vi "measurement_configurator.vi"() -> ()   [LabVIEW 2015]
doc: "Copyright (c) 2018 Frans Korhonen, Institute for Atmospheric and Earth System Research / Physics, Faculty of Science, University of Helsinki, Finland\n\nThis file is part of MeasGUI.\n\nThis Source Code Form is subject to the terms of the Mozilla Public\nLicense, v. 2.0. If a copy of the MPL was not distributed with this\n file, You can obtain one at http://mozilla.org/MPL/2.0/."
panel:
  in  "file cluster":T1={"open program folder"=FALSE, "Load"=FALSE, "Save"=FALSE, "Saved Configuration"="default", "output filename"="measurement.bat", "output"=FALSE}
  out "program path":path
  out "saved controls":string[](array[string])=["measurement channels", "measurement comments", "measurement parameters", "measurement settings", "measurement logging", "connection settings", "X channel", "Y channels", "Log x", "Log y", "save measurement", "measurement start commands", "measurement end commands"]
  in  "Tab Control":T2(tab)=enum."flowmeters"
  in  "serial device update rate":dbl=1.0
  in  "Serial devices":T3(array[cluster])
  in  "scaled output":T4(array[cluster])
  in  "scaled input":T5(array[cluster])
  in  "Electometer scaling":T6(array[cluster])
  in  "Concentration counters":T7(array[cluster])
  in  "TSI flowmeters":T8(array[cluster])
  in  "PID controllers":T9(array[cluster])
  in  "loggers":T10(array[cluster])
  in  "postconfiguration":string="#postconfiguration"
  in  "preconfiguration":string="create pipeserver pipe\nsetup pipe \"\\\\.\\pipe\\channel_system\"\nlink pipe control\n\nread control hardware.ini"
  out "configuration":string
  # "factor=current[A]/input"
  # "Will also create:\n\"channel_name\"_flow\n\"channel_name\"_t\n\"channel_name\"_p\n\nchannels for different measured parameters"
  # "Time specifiers in filenames \n%Y=year\n%m=Month as number\n%d = Day of the month\n%H =Hour in 24h format\n%M =Minute\n%S = seconds\n%z = Timezone offset"
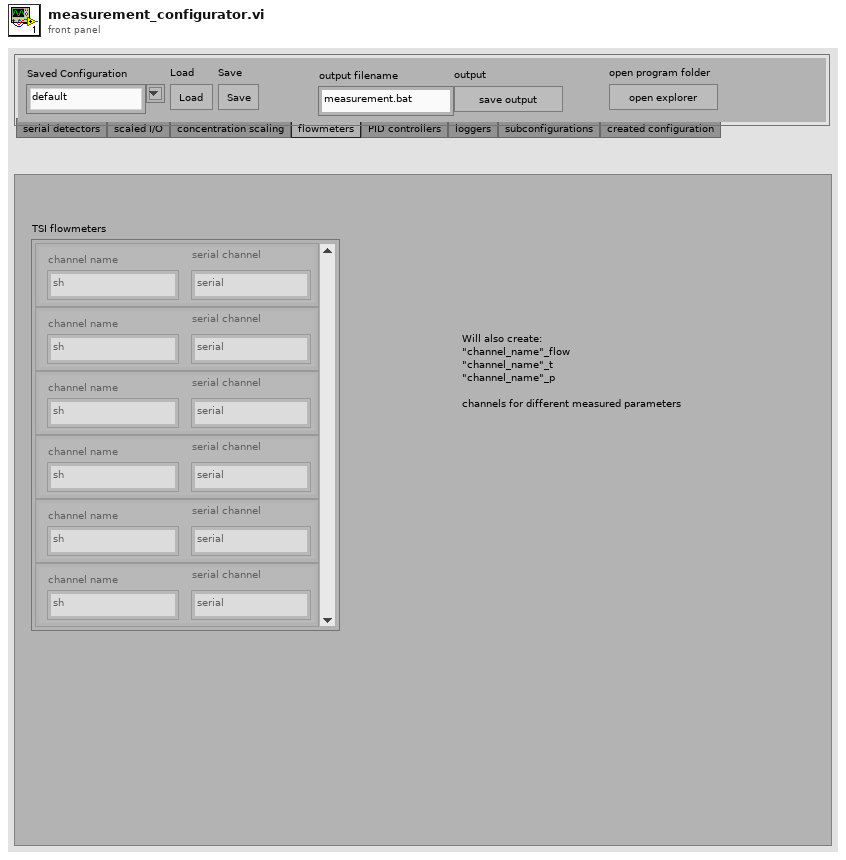
[diagram p1: front panel]
types:
  T1 = cluster{"open program folder":bool, "Load":bool, "Save":bool, "Saved Configuration":string, "output filename":string, "output":bool}
  T2 = enum32{"serial detectors", "scaled I/O", "concentration scaling", "flowmeters", "PID controllers", "loggers", "subconfigurations", "created configuration"}
  T3 = cluster{"channel name":string, "serial channel":string, "device":enum16{"Airmodus CPC", "TSI CPC", "TSI Electrometer", "Keithley EM", "TSI water CPC", "TSI CPC 3010"}}[]
  T4 = cluster{"channel name":string, "in 1":dbl, "output channel":string, "out 1":dbl, "in 2":dbl, "out 2":dbl}[]
  T5 = cluster{"channel name":string, "in 1":dbl, "input channel":string, "out 1":dbl, "in 2":dbl, "out 2":dbl}[]
  T6 = cluster{"channel name":string, "sample flow":dbl, "input channel":string, "factor":dbl, "input offset":dbl}[]
  T7 = cluster{"channel name":string, "sample flow":dbl, "counter input channel":string}[]
  T8 = cluster{"channel name":string, "serial channel":string}[]
  T9 = cluster{"channel name":string, "P":dbl, "input channel":string, "I":dbl, "in min":dbl, "in max":dbl, "out max":dbl, "out min":dbl, "initial sepoint":dbl, "D":dbl, "controlled channel":string}[]
  T10 = cluster{"channel name":string, "filename":string, "name change interval [s]":u32, "channels to log":string[], "delimiter char":string, "trigger char":string, "input channel\nor log interval [s]":string}[]
  T11 = enum16{"open", "replace", "create", "open or create", "replace or create", "replace or create with confirmation"}
  T12 = enum16{"Airmodus CPC", "TSI CPC", "TSI Electrometer", "Keithley EM", "TSI water CPC", "TSI CPC 3010"}
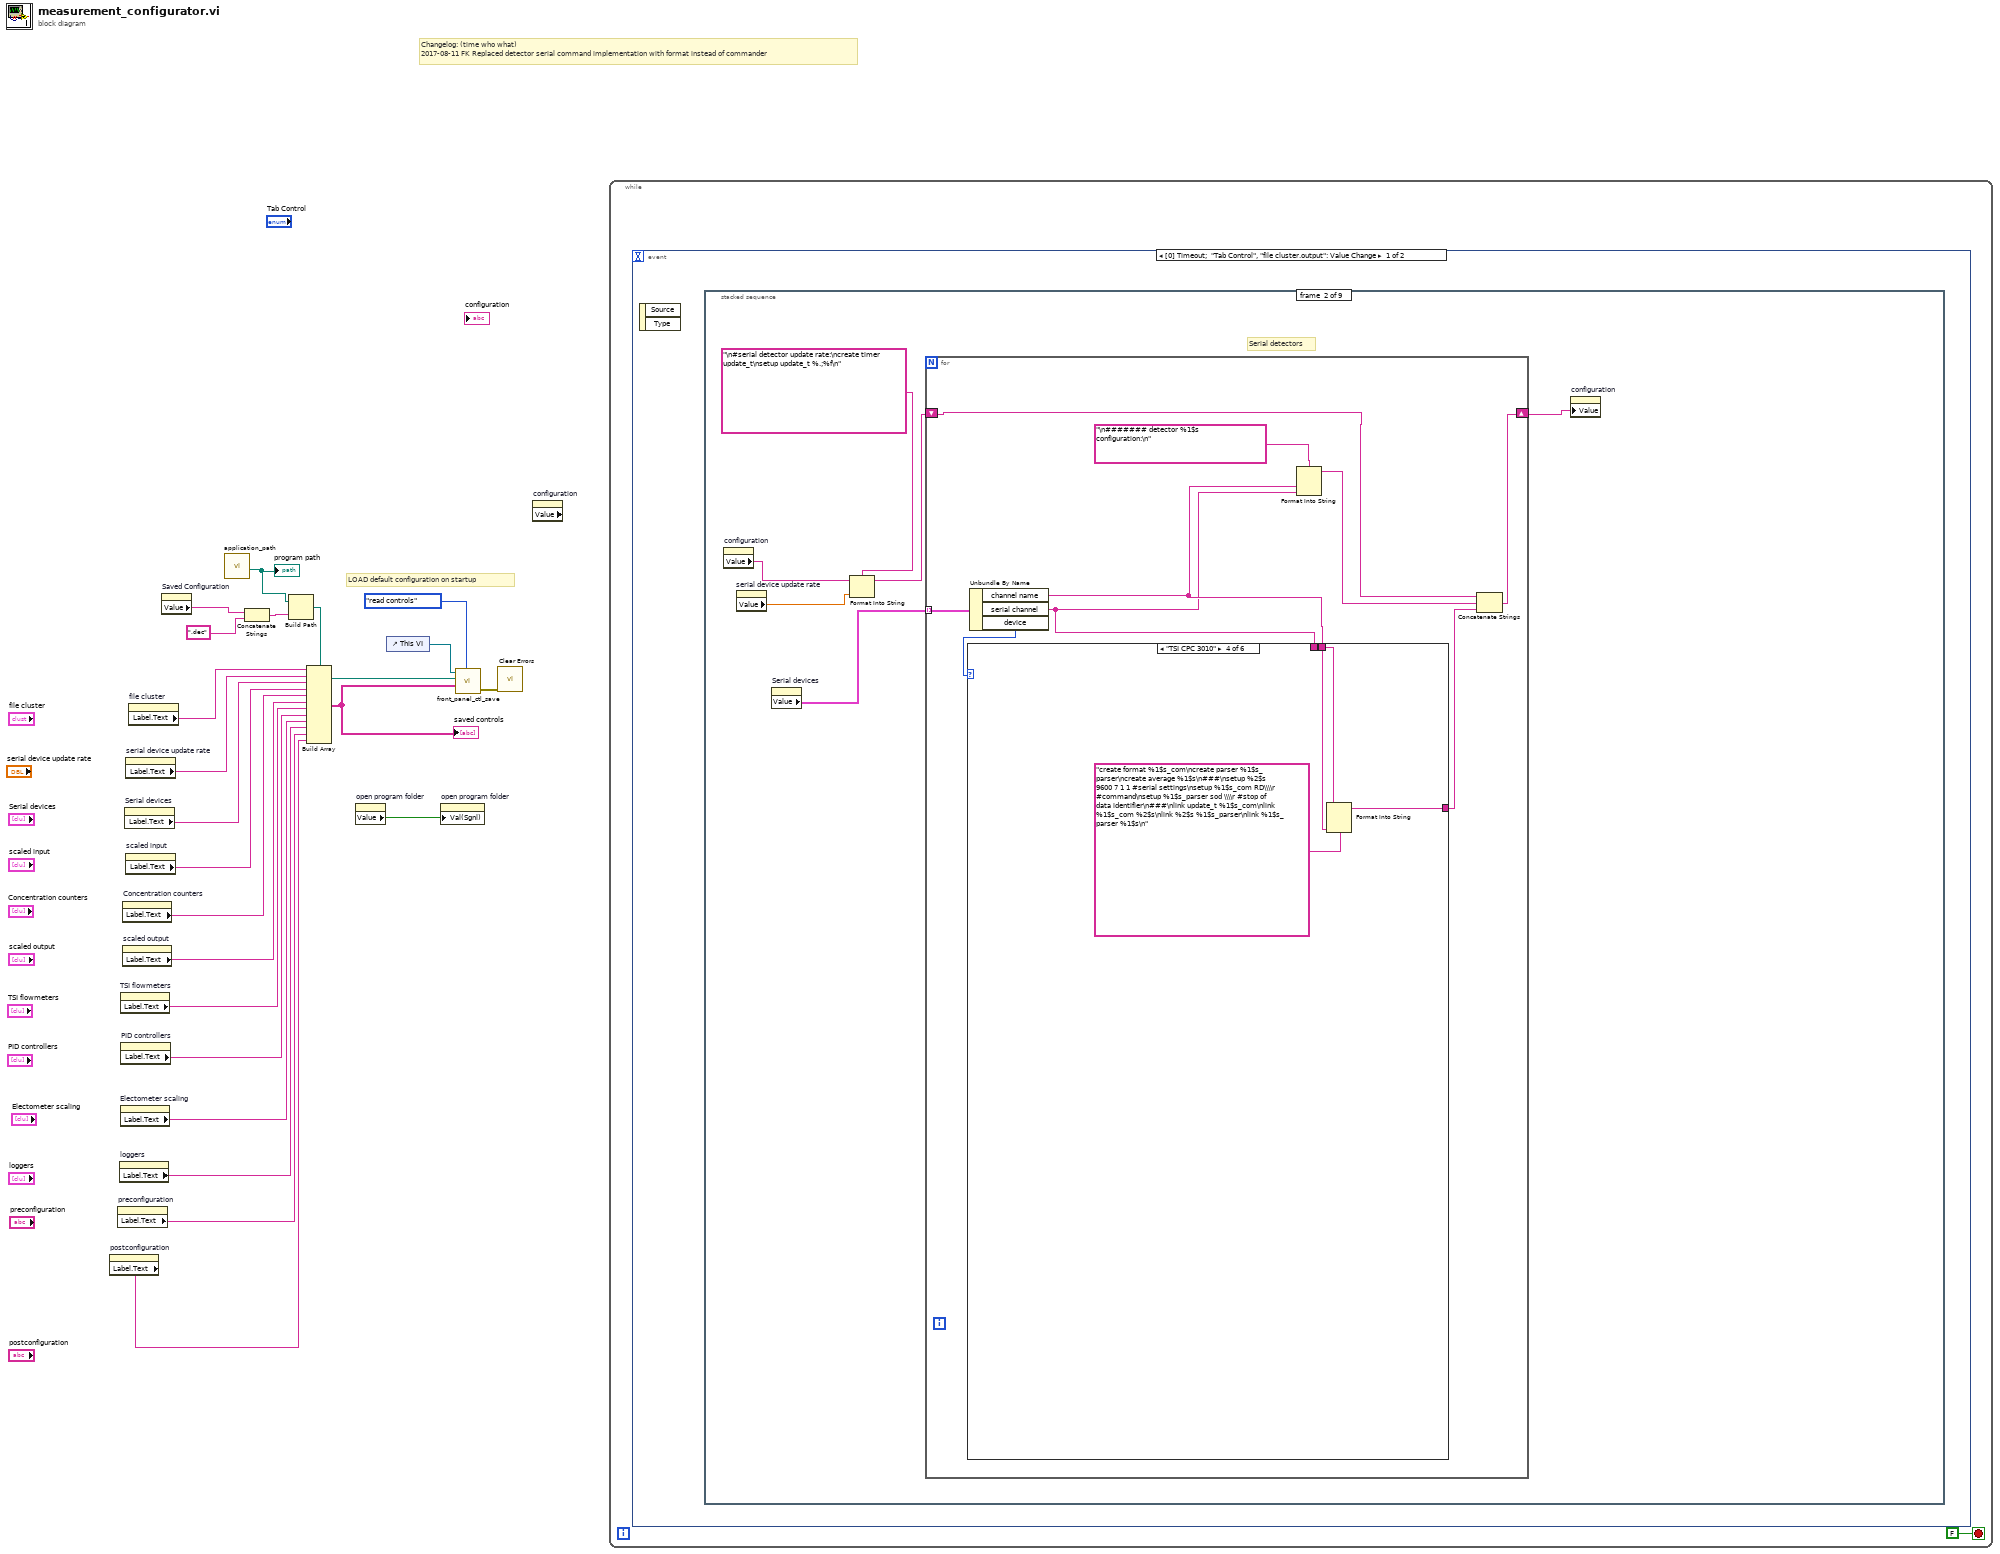
[diagram p0: block diagram]
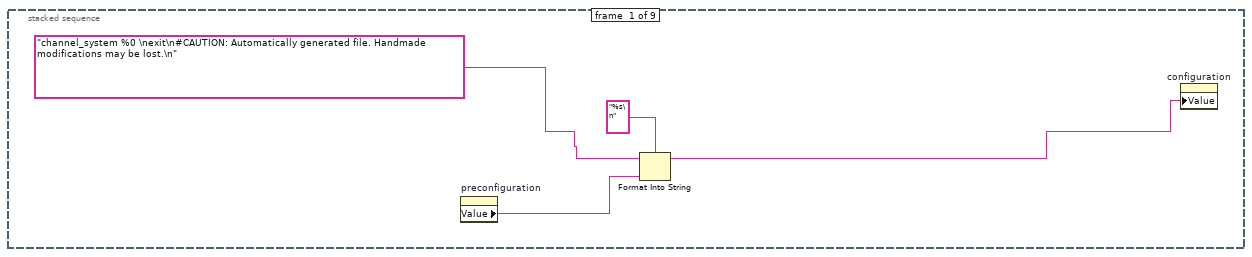
[diagram p2: hidden frame]
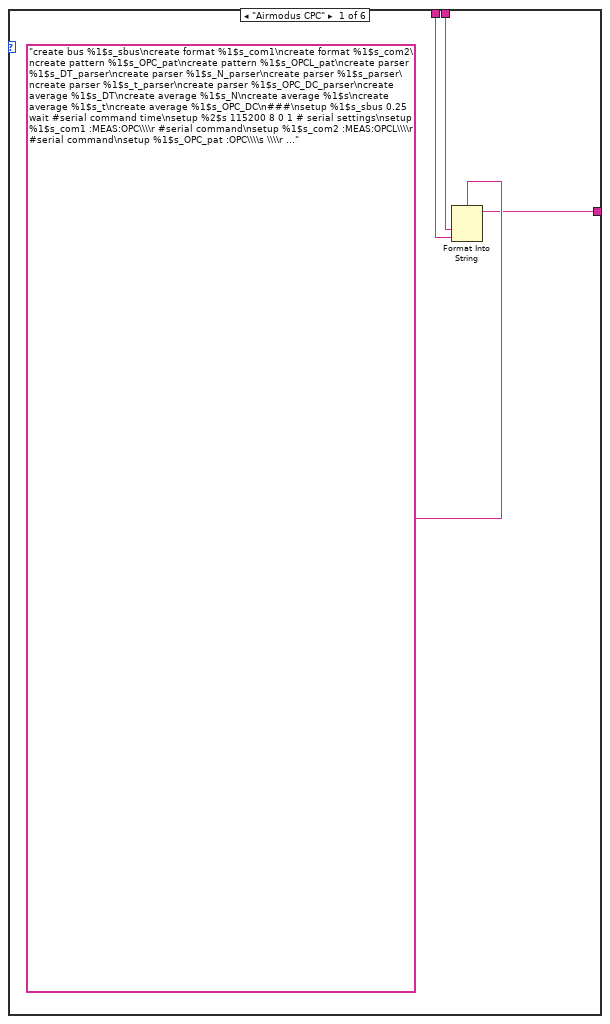
[diagram p3: hidden frame]
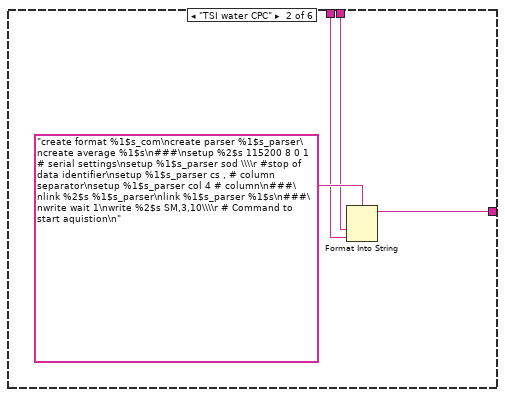
[diagram p4: hidden frame]
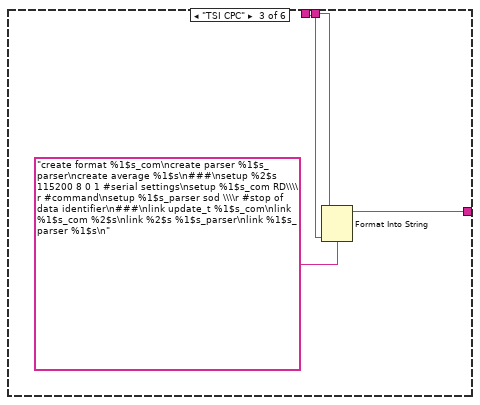
[diagram p5: hidden frame]
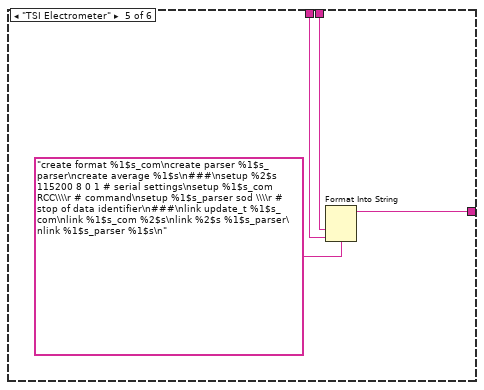
[diagram p6: hidden frame]
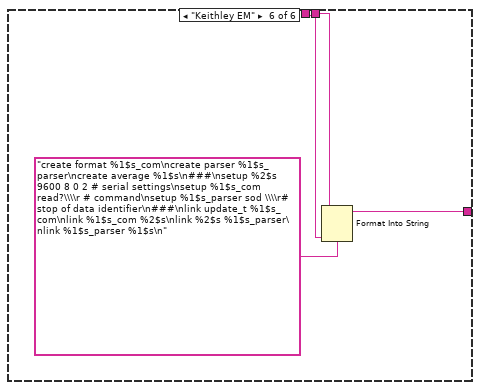
[diagram p7: hidden frame]
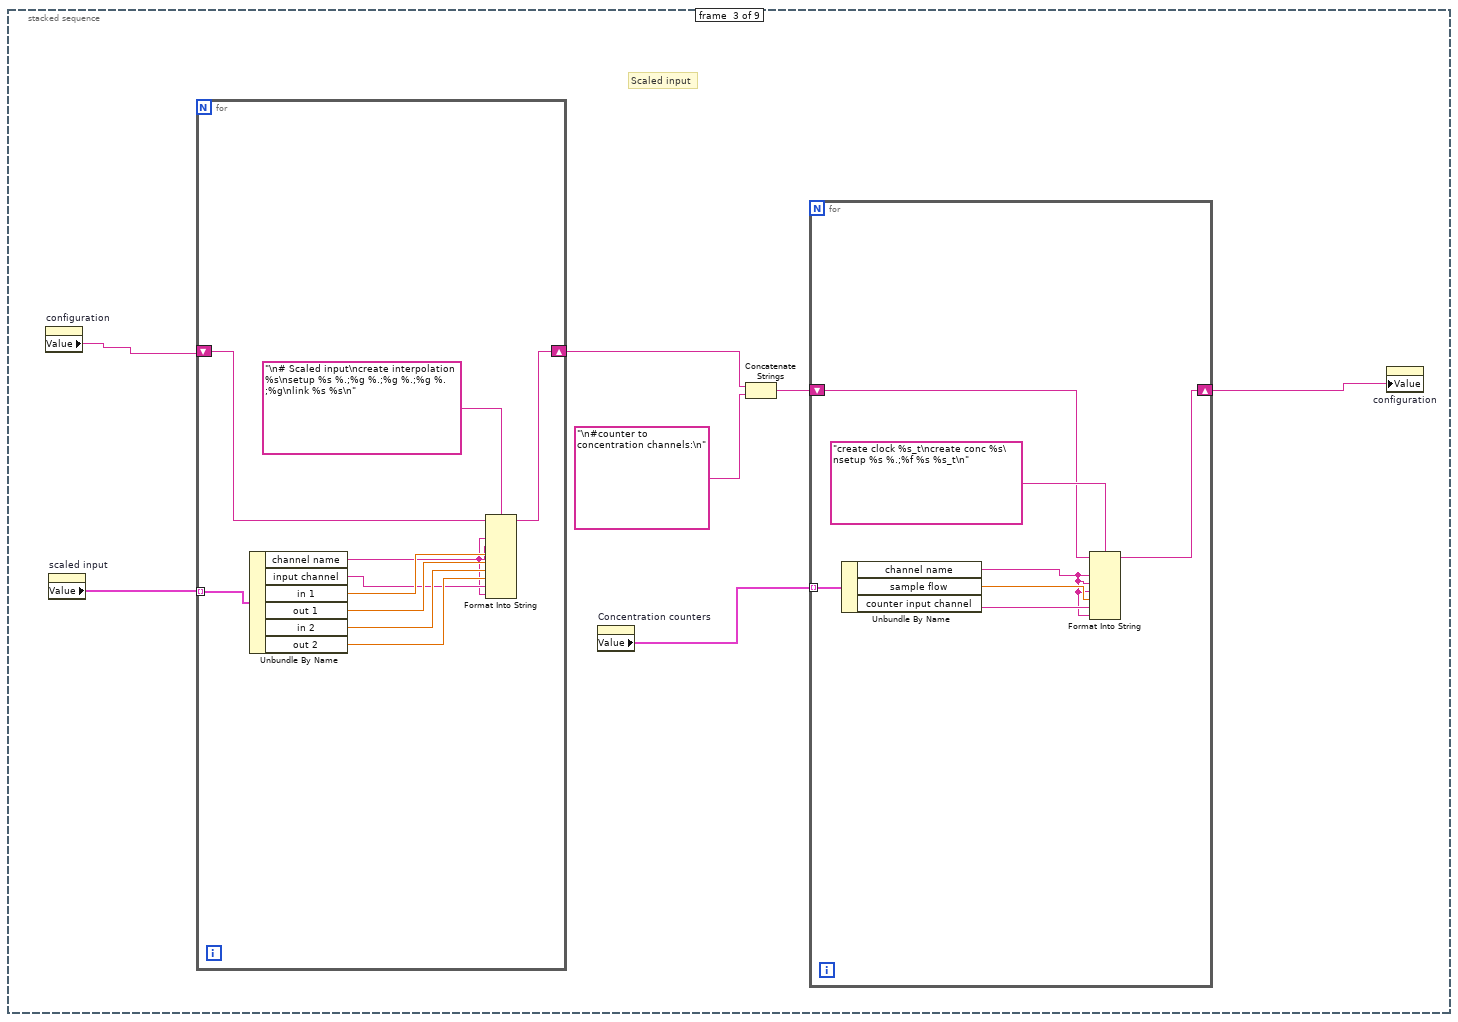
[diagram p8: hidden frame]
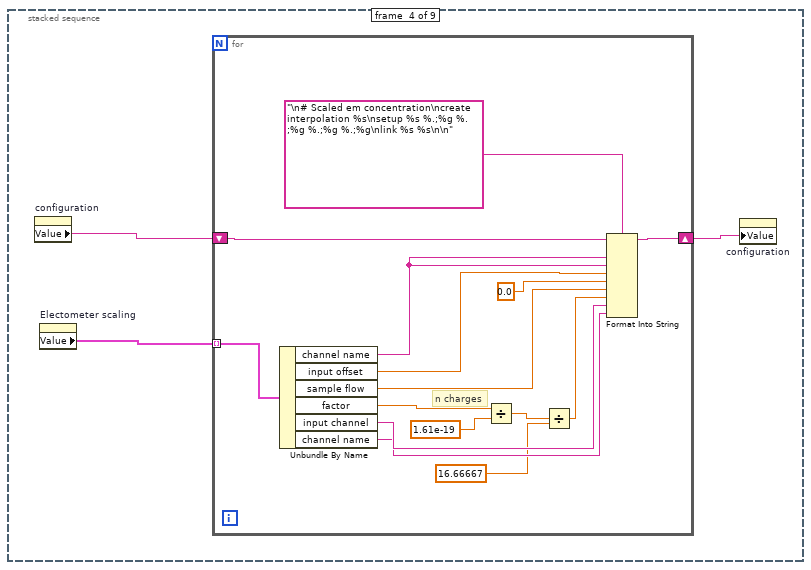
[diagram p9: hidden frame]
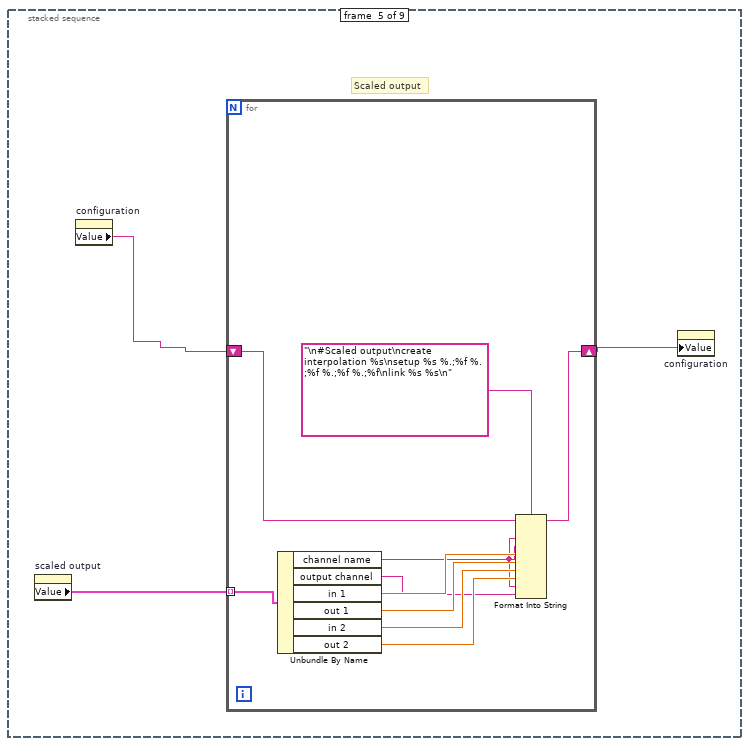
[diagram p10: hidden frame]
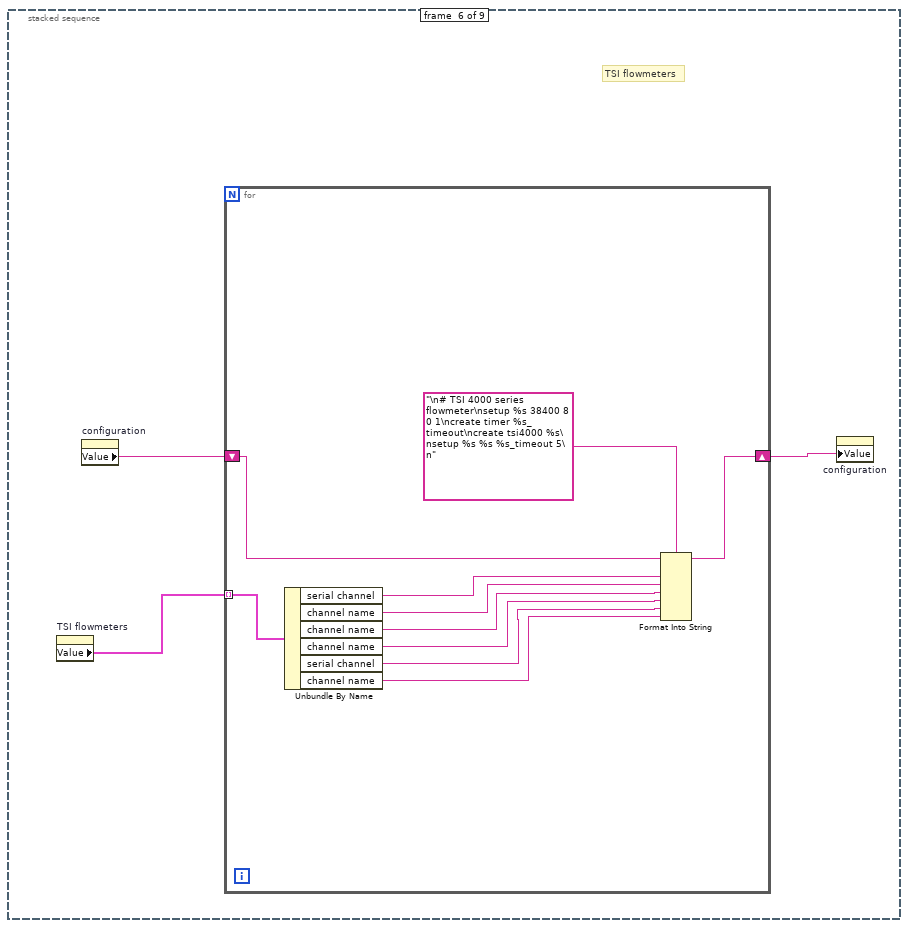
[diagram p11: hidden frame]
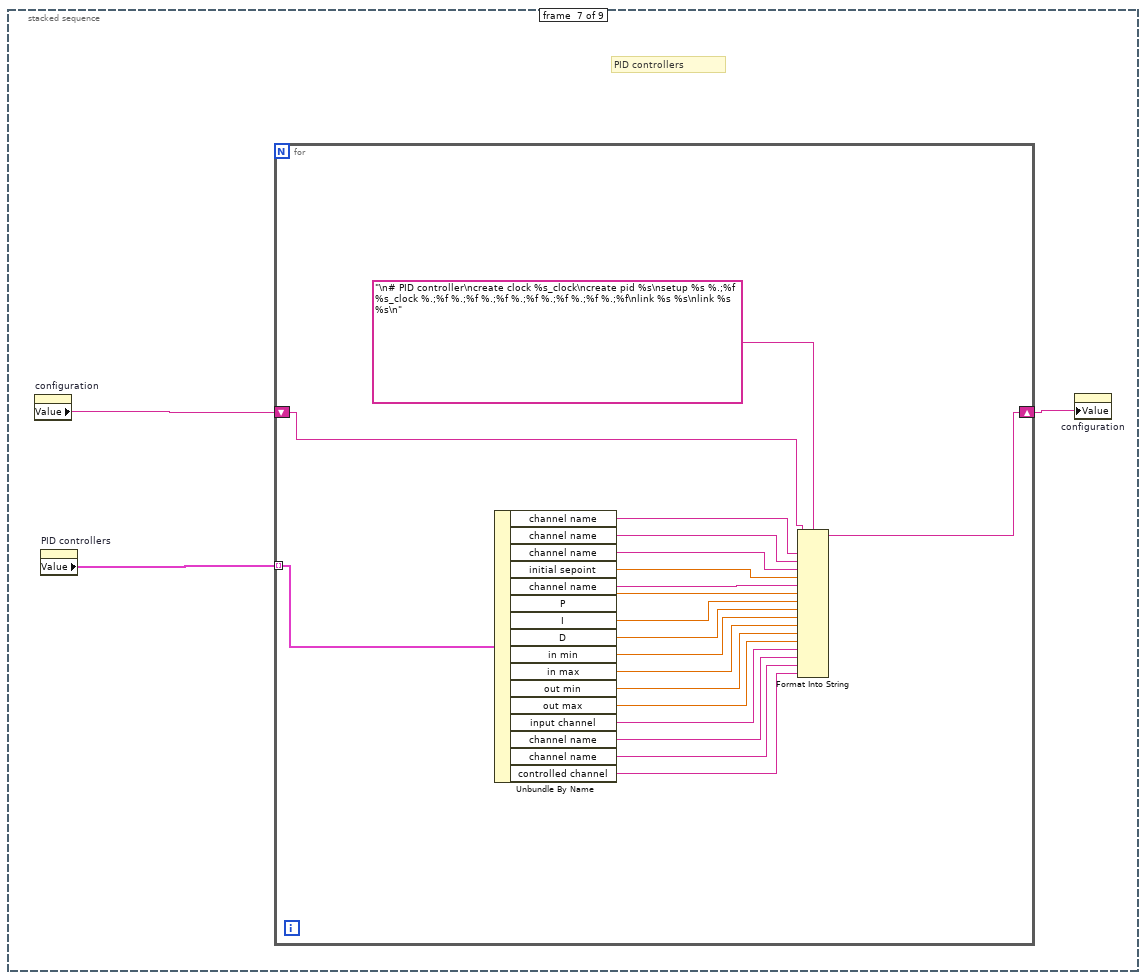
[diagram p12: hidden frame]
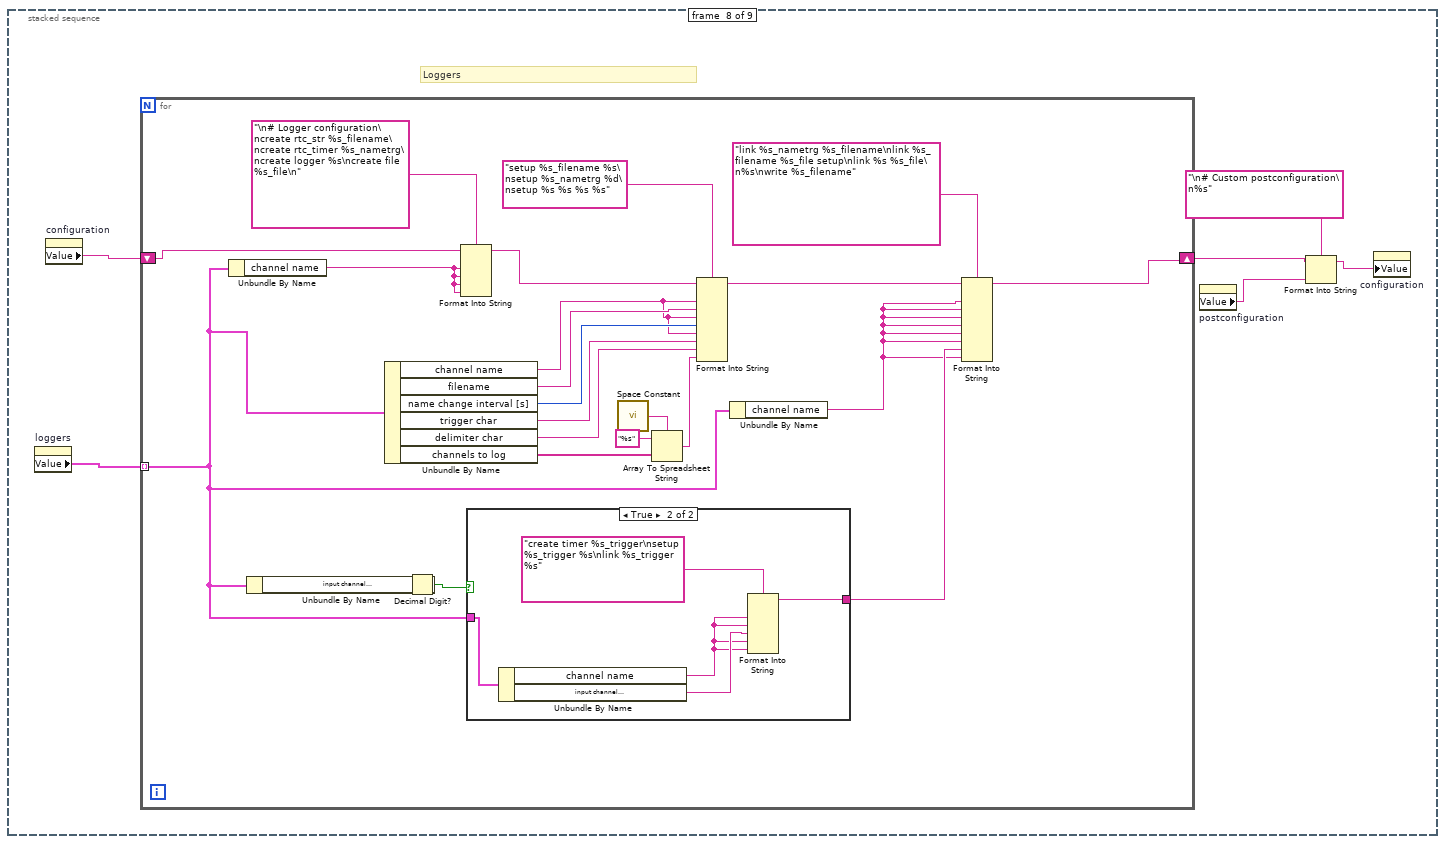
[diagram p13: hidden frame]
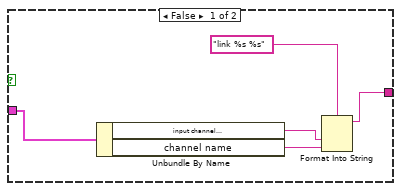
[diagram p14: hidden frame]
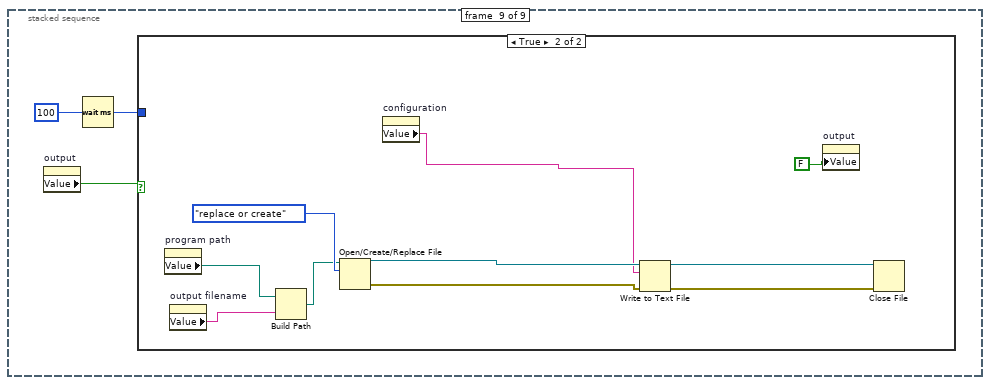
[diagram p15: hidden frame]
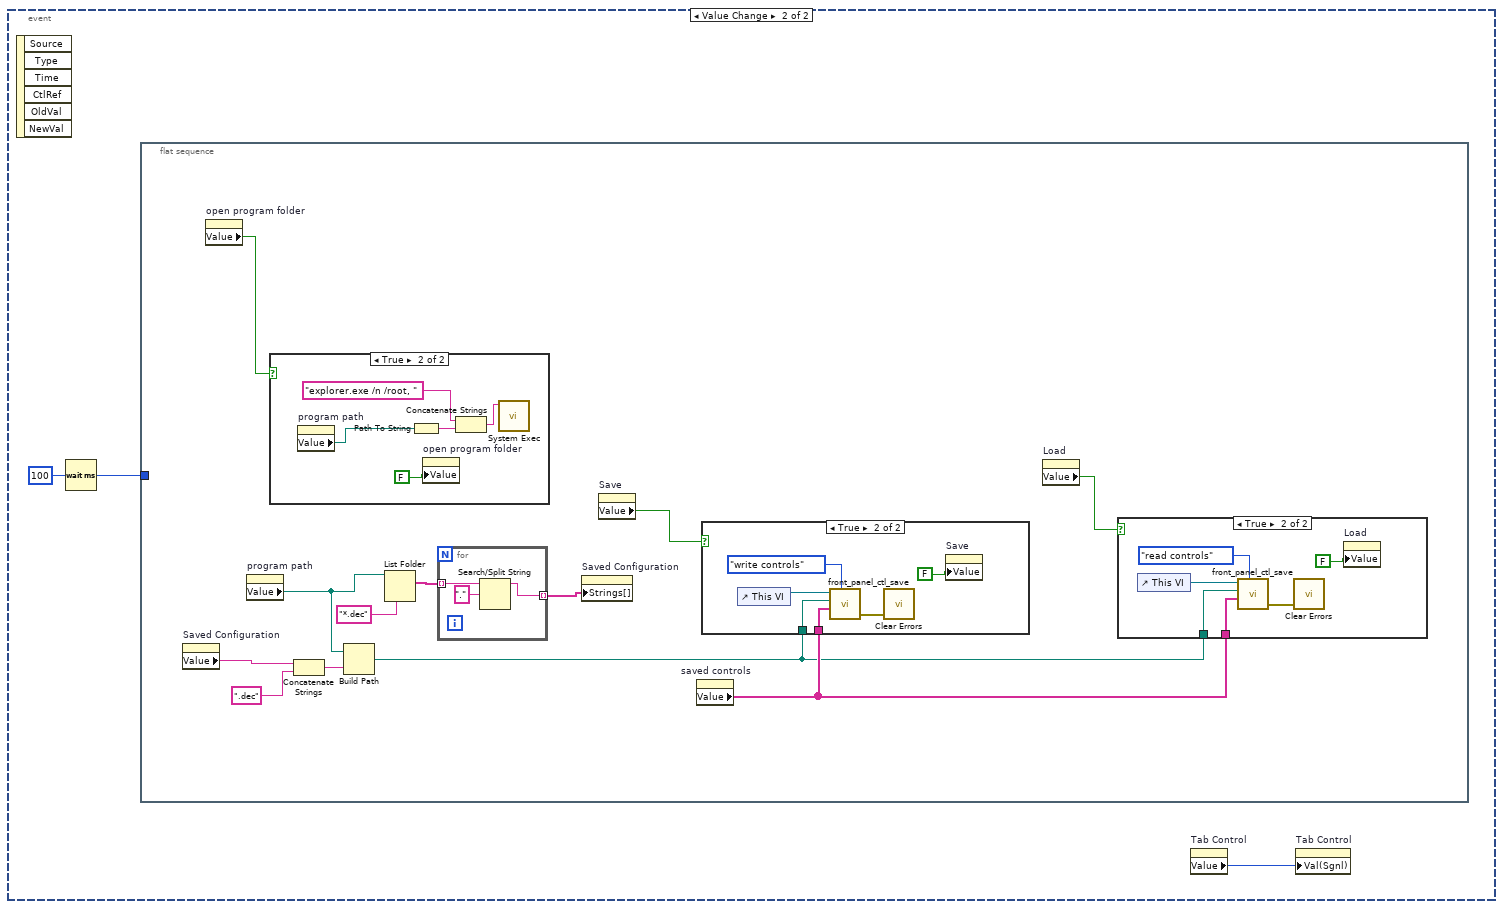
[diagram p17: hidden frame]
diagram:
  # "Changelog: (time who what)\n2017-08-11 FK Replaced detector serial command implementation with format instead of commander"
  # "LOAD default configuration on startup"
  n1 = property on="postconfiguration" class="Str"() -> ("Label.Text"=w1:string)  [unwired: 2 in, 2 out]
  n2 = property on="preconfiguration" class="Str"() -> ("Label.Text"=w2:string)  [unwired: 2 in, 2 out]
  n3 = property on="loggers" class="Arr (strict)"() -> ("Label.Text"=w4:string)  [unwired: 2 in, 2 out]
  n4 = property on="TSI flowmeters" class="Arr (strict)"() -> ("Label.Text"=w7:string)  [unwired: 2 in, 2 out]
  n5 = property on="Electometer scaling" class="Arr (strict)"() -> ("Label.Text"=w5:string)  [unwired: 2 in, 2 out]
  n6 = property on="PID controllers" class="Arr (strict)"() -> ("Label.Text"=w6:string)  [unwired: 2 in, 2 out]
  n7 = property on="Concentration counters" class="Arr (strict)"() -> ("Label.Text"=w12:string)  [unwired: 2 in, 2 out]
  n8 = property on="scaled output" class="Arr (strict)"() -> ("Label.Text"=w8:string)  [unwired: 2 in, 2 out]
  n9 = property on="Serial devices" class="Arr (strict)"() -> ("Label.Text"=w14:string)  [unwired: 2 in, 2 out]
  n10 = property on="serial device update rate" class="DigNum (strict)"() -> ("Label.Text"=w15:string)  [unwired: 2 in, 2 out]
  n11 = property on="scaled input" class="Arr (strict)"() -> ("Label.Text"=w13:string)  [unwired: 2 in, 2 out]
  n12 = property on="file cluster" class="Clust (strict)"() -> ("Label.Text"=w11:string)  [unwired: 2 in, 2 out]
  n13 = property on="Saved Configuration" class="CmbBox"() -> ("Value"=w17:string)  [unwired: 2 in, 2 out]
  n14 = call "application_path.vi"() -> ("path"=w10:path)  [unwired: 11 in]
  "program path" <- w10
  n15 = Concatenate Strings(w17, ".dec" ("string")) -> (w21:string)
  n16 = Build Path(base path=w10, name or relative path=w21) -> (appended path=w19:path)
  n17 = Build Array(w11, w15, w14, w13, w12, w8, w7, w6, w5, w4, w2, w1) -> (w16:string[])
  "saved controls" <- w16
  n18 = property on="open program folder" class="Bool (strict)"() -> ("Value"=w9:bool)  [unwired: 2 in, 2 out]
  n19 = control-ref of="This VI"() -> (w18:refnum<vi>)
  n20 = property on="open program folder" class="Bool (strict)"("Val(Sgnl)"=w9) -> ()  [unwired: 2 in, 2 out]
  n21 = call "front_panel_ctl_save.vi"("VI in"=w18, "method"=enum16{"read controls", "write controls"}."read controls", "filename"=w19, "controls"=w16) -> ("error out"=w3:errorcluster)  [unwired: 4 in]
  n22 = call <vilib>:"Clear Errors.vi"("error in (no error)"=w3) -> ()  [unwired: 5 in, 2 out]
  n23 = property on="configuration" class="Str" props=["Value"]() -> ()  [unwired: 2 in, 3 out]
  n24 = while {
    stop <- FALSE stop-if-true
    n25 = event shown="[0] Timeout;  \"Tab Control\", \"file cluster.output\": Value Change" {
      selector: _ -> [_ _]
      dyn-events: _ -> [_ _]
      timeout: _ -> [_ _]
      event Timeout; "Tab Control", "file cluster.output": Value Change {
        n26 = event-data() -> ()  [unwired: 1 in, 2 out]
        n27 = stacked-sequence {
          frame #0 {
            n28 = property on="preconfiguration" class="Str"() -> ("Value"=w27:string)  [unwired: 2 in, 2 out]
            n29 = Format Into String(format string="%s\n", initial string="channel_system %0 \nexit\n#CAUTION: Automatically generated file. Handmade modifications may be lost.\n", w27) -> (resulting string=w26:string)  [unwired: 1 in, 1 out]
            n30 = property on="configuration" class="Str"("Value"=w26) -> ()  [unwired: 2 in, 2 out]
          }
          frame #1 {
            # "Serial detectors"
            n31 = property on="configuration" class="Str"() -> ("Value"=w28:string)  [unwired: 2 in, 2 out]
            n32 = property on="serial device update rate" class="DigNum (strict)"() -> ("Value"=w29:dbl)  [unwired: 2 in, 2 out]
            n33 = property on="Serial devices" class="Arr (strict)"() -> ("Value"=w32:T3)  [unwired: 2 in, 2 out]
            n34 = Format Into String(format string="\n#serial detector update rate:\ncreate timer update_t\nsetup update_t %.;%f\n", initial string=w28, w29) -> (resulting string=w30:string)  [unwired: 1 in, 1 out]
            n35 = for {
              tunnel: w32 -> [w42] mode=indexing
              shift-right: [w38] -> w33
              shift-left: w30 -> [w37]
              n36 = Unbundle By Name(w42) -> ("channel name"=w35:string, "serial channel"=w34:string, "device"=w36:T12)
              n37 = case shown="\"TSI CPC 3010\"" w36 {
                tunnel: w34 -> [w43 w47 w51 w55 w59 w63]
                tunnel: [w45 w50 w53 w57 w61 w65] -> w39
                tunnel: w35 -> [w44 w48 w52 w56 w60 w64]
                frame "Airmodus CPC" {
                  n38 = Format Into String(format string="create bus %1$s_sbus\ncreate format %1$s_com1\ncreate format %1$s_com2\ncreate pattern %1$s_OPC_pat\ncreate pattern %1$s_OPCL_pat\ncreate parser %1$s_DT_parser\ncreate parser %1$s_N_parser\ncreate parser %1$s_parser\ncreate parser %1$s_t_parser\ncreate parser %1$s_OPC_DC_parser\ncreate average %1$s_DT\ncreate average %1$s_N\ncreate average %1$s\ncreate average %1$s_t\ncreate average %1$s_OPC_DC\n###\nsetup %1$s_sbus 0.25 wait #serial command time\nsetup %2$s 115200 8 0 1 # serial settings\nsetup %1$s_com1 :MEAS:OPC\\\\r #serial command\nsetup %1$s_com2 :MEAS:OPCL\\\\r  #serial command\nsetup %1$s_OPC_pat :OPC\\\\s \\\\r 256\nsetup %1$s_OPCL_pat :OPCL\\\\s \\\\r 256\n###\nsetup %1$s_DT_parser sod \\\\r #stop of data identifier\nsetup %1$s_DT_parser cs , # column separator\nsetup %1$s_DT_parser col 0 # column\n###\nsetup %1$s_N_parser sod \\\\r #stop of data identifier\nsetup %1$s_N_parser cs , # column separator\nsetup %1$s_N_parser col 1 # column\n###\nsetup %1$s_parser sod \\\\r #stop of data identifier\nsetup %1$s_parser cs , # column separator\nsetup %1$s_parser col 2 # column\n###\nsetup %1$s_t_parser sod \\\\r #stop of data identifier\nsetup %1$s_t_parser cs , # column separator\nsetup %1$s_t_parser col 3 # column\n###\nsetup %1$s_OPC_DC_parser sod \\\\r #stop of data identifier\nsetup %1$s_OPC_DC_parser cs , #column separator\nsetup %1$s_OPC_DC_parser col 0 #column\n###\nlink update_t %1$s_com1\nlink update_t %1$s_com2\nlink %1$s_com1 %1$s_sbus\nlink %1$s_com2 %1$s_sbus\nlink %1$s_sbus %2$s\nlink %2$s %1$s_OPC_pat\nlink %2$s %1$s_OPCL_pat\n###\nlink %1$s_OPC_pat %1$s_DT_parser\nlink %1$s_OPC_pat %1$s_N_parser\nlink %1$s_OPC_pat %1$s_parser\nlink %1$s_OPC_pat %1$s_t_parser\nlink %1$s_OPCL_pat %1$s_OPC_DC_parser\n###\nlink %1$s_DT_parser  %1$s_DT\nlink %1$s_N_parser %1$s_N\nlink %1$s_parser %1$s\nlink %1$s_t_parser %1$s_t\nlink %1$s_OPC_DC_parser %1$s_OPC_DC\n", w44, w43) -> (resulting string=w45:string)  [unwired: 2 in, 1 out]
                }
                frame "TSI water CPC" {
                  n39 = Format Into String(format string="create format %1$s_com\ncreate parser %1$s_parser\ncreate average %1$s\n###\nsetup %2$s 115200 8 0 1 # serial settings\nsetup %1$s_parser sod \\\\r #stop of data identifier\nsetup %1$s_parser cs , # column separator\nsetup %1$s_parser col 4 # column\n###\nlink %2$s %1$s_parser\nlink %1$s_parser %1$s\n###\nwrite wait 1\nwrite %2$s SM,3,10\\\\r # Command to start aquistion\n", w48, w47) -> (resulting string=w50:string)  [unwired: 2 in, 1 out]
                }
                frame "TSI CPC" {
                  n40 = Format Into String(format string="create format %1$s_com\ncreate parser %1$s_parser\ncreate average %1$s\n###\nsetup %2$s 115200 8 0 1 #serial settings\nsetup %1$s_com RD\\\\r #command\nsetup %1$s_parser sod \\\\r #stop of data identifier\n###\nlink update_t %1$s_com\nlink %1$s_com %2$s\nlink %2$s %1$s_parser\nlink %1$s_parser %1$s\n", w52, w51) -> (resulting string=w53:string)  [unwired: 2 in, 1 out]
                }
                frame "TSI CPC 3010" {
                  n41 = Format Into String(format string="create format %1$s_com\ncreate parser %1$s_parser\ncreate average %1$s\n###\nsetup %2$s 9600 7 1 1 #serial settings\nsetup %1$s_com RD\\\\r #command\nsetup %1$s_parser sod \\\\r #stop of data identifier\n###\nlink update_t %1$s_com\nlink %1$s_com %2$s\nlink %2$s %1$s_parser\nlink %1$s_parser %1$s\n", w56, w55) -> (resulting string=w57:string)  [unwired: 2 in, 1 out]
                }
                frame "TSI Electrometer" {
                  n42 = Format Into String(format string="create format %1$s_com\ncreate parser %1$s_parser\ncreate average %1$s\n###\nsetup %2$s 115200 8 0 1 # serial settings\nsetup %1$s_com RCC\\\\r # command\nsetup %1$s_parser sod \\\\r # stop of data identifier\n###\nlink update_t %1$s_com\nlink %1$s_com %2$s\nlink %2$s %1$s_parser\nlink %1$s_parser %1$s\n", w60, w59) -> (resulting string=w61:string)  [unwired: 2 in, 1 out]
                }
                frame "Keithley EM" {
                  n43 = Format Into String(format string="create format %1$s_com\ncreate parser %1$s_parser\ncreate average %1$s\n###\nsetup %2$s 9600 8 0 2 # serial settings\nsetup %1$s_com read?\\\\r # command\nsetup %1$s_parser sod \\\\r# stop of data identifier\n###\nlink update_t %1$s_com\nlink %1$s_com %2$s\nlink %2$s %1$s_parser\nlink %1$s_parser %1$s\n", w64, w63) -> (resulting string=w65:string)  [unwired: 2 in, 1 out]
                }
              }
              n44 = Format Into String(format string="\n####### detector %1$s configuration:\n", w35, w34) -> (resulting string=w40:string)  [unwired: 2 in, 1 out]
              n45 = Concatenate Strings(w37, w40, w39) -> (w38:string)
            }
            n46 = property on="configuration" class="Str"("Value"=w33) -> ()  [unwired: 2 in, 2 out]
          }
          frame #2 {
            # "Scaled input"
            n47 = property on="configuration" class="Str"() -> ("Value"=w67:string)  [unwired: 2 in, 2 out]
            n48 = property on="scaled input" class="Arr (strict)"() -> ("Value"=w69:T5)  [unwired: 2 in, 2 out]
            n49 = for {
              tunnel: w69 -> [w90] mode=indexing
              shift-right: [w81] -> w73
              shift-left: w67 -> [w82]
              n50 = Unbundle By Name(w90) -> ("channel name"=w83:string, "input channel"=w84:string, "in 1"=w88:dbl, "out 1"=w87:dbl, "in 2"=w86:dbl, "out 2"=w85:dbl)
              n51 = Format Into String(format string="\n# Scaled input\ncreate interpolation %s\nsetup %s %.;%g %.;%g %.;%g %.;%g\nlink %s %s\n", initial string=w82, w83, w83, w88, w87, w86, w85, w84, w83) -> (resulting string=w81:string)  [unwired: 1 in, 1 out]
            }
            n52 = property on="Concentration counters" class="Arr (strict)"() -> ("Value"=w68:T7)  [unwired: 2 in, 2 out]
            n53 = Concatenate Strings(w73, "\n#counter to concentration channels:\n" ("format string")) -> (w71:string)
            n54 = for {
              tunnel: w68 -> [w80] mode=indexing
              shift-right: [w76] -> w70
              shift-left: w71 -> [w75]
              n55 = Unbundle By Name(w80) -> ("channel name"=w74:string, "sample flow"=w78:dbl, "counter input channel"=w77:string)
              n56 = Format Into String(format string="create clock %s_t\ncreate conc %s\nsetup %s %.;%f %s %s_t\n", initial string=w75, w74, w74, w74, w78, w77, w74) -> (resulting string=w76:string)  [unwired: 1 in, 1 out]
            }
            n57 = property on="configuration" class="Str"("Value"=w70) -> ()  [unwired: 2 in, 2 out]
          }
          frame #3 {
            n58 = property on="configuration" class="Str"() -> ("Value"=w92:string)  [unwired: 2 in, 2 out]
            n59 = property on="Electometer scaling" class="Arr (strict)"() -> ("Value"=w93:T6)  [unwired: 2 in, 2 out]
            n60 = for {
              tunnel: w93 -> [w108] mode=indexing
              shift-right: [w103] -> w91
              shift-left: w92 -> [w104]
              # "n charges"
              n61 = Unbundle By Name(w108) -> ("channel name"=w99:string, "input offset"=w100:dbl, "sample flow"=w102:dbl, "factor"=w107:dbl, "input channel"=w98:string, "channel name"=w97:string)
              n62 = Divide(x=w107, y=1.61e-19) -> (x/y=w95:dbl)
              n63 = Divide(x=w95, y=16.66667) -> (x/y=w94:dbl)
              n64 = Format Into String(format string="\n# Scaled em concentration\ncreate interpolation %s\nsetup %s %.;%g %.;%g %.;%g %.;%g\nlink %s %s\n\n", initial string=w104, w99, w99, w100, 0.0 ("input 4"), w102, w94, w98, w97) -> (resulting string=w103:string)  [unwired: 1 in, 1 out]
            }
            n65 = property on="configuration" class="Str"("Value"=w91) -> ()  [unwired: 2 in, 2 out]
          }
          frame #4 {
            # "Scaled output"
            n66 = property on="scaled output" class="Arr (strict)"() -> ("Value"=w111:T4)  [unwired: 2 in, 2 out]
            n67 = property on="configuration" class="Str"() -> ("Value"=w109:string)  [unwired: 2 in, 2 out]
            n68 = for {
              tunnel: w111 -> [w121] mode=indexing
              shift-right: [w114] -> w110
              shift-left: w109 -> [w115]
              n69 = Unbundle By Name(w121) -> ("channel name"=w113:string, "output channel"=w112:string, "in 1"=w119:dbl, "out 1"=w118:dbl, "in 2"=w117:dbl, "out 2"=w116:dbl)
              n70 = Format Into String(format string="\n#Scaled output\ncreate interpolation %s\nsetup %s %.;%f %.;%f %.;%f %.;%f\nlink %s %s\n", initial string=w115, w113, w113, w119, w118, w117, w116, w113, w112) -> (resulting string=w114:string)  [unwired: 1 in, 1 out]
            }
            n71 = property on="configuration" class="Str"("Value"=w110) -> ()  [unwired: 2 in, 2 out]
          }
          frame #5 {
            # "TSI flowmeters"
            n72 = property on="TSI flowmeters" class="Arr (strict)"() -> ("Value"=w122:T8)  [unwired: 2 in, 2 out]
            n73 = property on="configuration" class="Str"() -> ("Value"=w124:string)  [unwired: 2 in, 2 out]
            n74 = for {
              tunnel: w122 -> [w133] mode=indexing
              shift-right: [w131] -> w123
              shift-left: w124 -> [w132]
              n75 = Unbundle By Name(w133) -> ("serial channel"=w130:string, "channel name"=w129:string, "channel name"=w128:string, "channel name"=w127:string, "serial channel"=w126:string, "channel name"=w125:string)
              n76 = Format Into String(format string="\n# TSI 4000 series flowmeter\nsetup %s 38400 8 0 1\ncreate timer %s_timeout\ncreate tsi4000 %s\nsetup %s %s %s_timeout 5\n", initial string=w132, w130, w129, w128, w127, w126, w125) -> (resulting string=w131:string)  [unwired: 1 in, 1 out]
            }
            n77 = property on="configuration" class="Str"("Value"=w123) -> ()  [unwired: 2 in, 2 out]
          }
          frame #6 {
            # "PID controllers"
            n78 = property on="configuration" class="Str"() -> ("Value"=w137:string)  [unwired: 2 in, 2 out]
            n79 = property on="PID controllers" class="Arr (strict)"() -> ("Value"=w135:T9)  [unwired: 2 in, 2 out]
            n80 = for {
              tunnel: w135 -> [w157] mode=indexing
              shift-right: [w139] -> w136
              shift-left: w137 -> [w138]
              n81 = Unbundle By Name(w157) -> ("channel name"=w155:string, "channel name"=w154:string, "channel name"=w153:string, "initial sepoint"=w152:dbl, "channel name"=w151:string, "P"=w150:dbl, "I"=w149:dbl, "D"=w148:dbl, "in min"=w147:dbl, "in max"=w146:dbl, "out min"=w145:dbl, "out max"=w144:dbl, "input channel"=w143:string, "channel name"=w142:string, "channel name"=w141:string, "controlled channel"=w140:string)
              n82 = Format Into String(format string="\n# PID controller\ncreate clock %s_clock\ncreate pid %s\nsetup %s %.;%f %s_clock %.;%f %.;%f %.;%f %.;%f %.;%f %.;%f %.;%f\nlink %s %s\nlink %s %s\n", initial string=w138, w155, w154, w153, w152, w151, w150, w149, w148, w147, w146, w145, w144, w143, w142, w141, w140) -> (resulting string=w139:string)  [unwired: 1 in, 1 out]
            }
            n83 = property on="configuration" class="Str"("Value"=w136) -> ()  [unwired: 2 in, 2 out]
          }
          frame #7 {
            # "Loggers"
            n84 = property on="loggers" class="Arr (strict)"() -> ("Value"=w162:T10)  [unwired: 2 in, 2 out]
            n85 = property on="configuration" class="Str"() -> ("Value"=w163:string)  [unwired: 2 in, 2 out]
            n86 = for {
              shift-right: [w164] -> w161
              shift-left: w163 -> [w171]
              tunnel: w162 -> [w167] mode=indexing
              n87 = Unbundle By Name(w167) -> ("channel name"=w182:string)
              n88 = Unbundle By Name(w167) -> ("input channel\nor log interval [s]"=w183:string)
              n89 = Unbundle By Name(w167) -> ("channel name"=w170:string, "filename"=w177:string, "name change interval [s]"=w176:u32, "trigger char"=w175:string, "delimiter char"=w174:string, "channels to log"=w173:string[])
              n90 = Decimal Digit?(1:w183) -> (0:w184:bool)
              n91 = Format Into String(format string="\n# Logger configuration\ncreate rtc_str %s_filename\ncreate rtc_timer %s_nametrg\ncreate logger %s\ncreate file %s_file\n", initial string=w171, w182, w182, w182, w182) -> (resulting string=w178:string)  [unwired: 1 in, 1 out]
              n92 = case shown="True" w184 {
                tunnel: w167 -> [w188 w195]
                tunnel: [w189 w191] -> w166
                frame False {
                  n93 = Unbundle By Name(w188) -> ("input channel\nor log interval [s]"=w187:string, "channel name"=w186:string)
                  n94 = Format Into String(format string="link %s %s", w187, w186) -> (resulting string=w189:string)  [unwired: 2 in, 1 out]
                }
                frame True {
                  n95 = Unbundle By Name(w195) -> ("channel name"=w192:string, "input channel\nor log interval [s]"=w193:string)
                  n96 = Format Into String(format string="create timer %s_trigger\nsetup %s_trigger %s\nlink %s_trigger %s", w192, w192, w193, w192, w192) -> (resulting string=w191:string)  [unwired: 2 in, 1 out]
                }
              }
              n97 = call <vilib>:"Space Constant.vi"() -> ("String"=w181:string)
              n98 = Array To Spreadsheet String(delimiter (Tab)=w181, array=w173, 3:"%s" ("format string")) -> (spreadsheet string=w172:string)
              n99 = Format Into String(format string="setup %s_filename %s\nsetup %s_nametrg %d\nsetup %s %s %s %s", initial string=w178, w170, w177, w170, w176, w170, w175, w174, w172) -> (resulting string=w169:string)  [unwired: 1 in, 1 out]
              n100 = Unbundle By Name(w167) -> ("channel name"=w165:string)
              n101 = Format Into String(format string="link %s_nametrg %s_filename\nlink %s_filename %s_file setup\nlink %s %s_file\n%s\nwrite %s_filename", initial string=w169, w165, w165, w165, w165, w165, w165, w166, w165) -> (resulting string=w164:string)  [unwired: 1 in, 1 out]
            }
            n102 = property on="postconfiguration" class="Str"() -> ("Value"=w159:string)  [unwired: 2 in, 2 out]
            n103 = Format Into String(format string="\n# Custom postconfiguration\n%s", initial string=w161, w159) -> (resulting string=w160:string)  [unwired: 1 in, 1 out]
            n104 = property on="configuration" class="Str"("Value"=w160) -> ()  [unwired: 2 in, 2 out]
          }
          frame #8 {
            n105 = property on="output" class="Bool (strict)"() -> ("Value"=w198:bool)  [unwired: 2 in, 2 out]
            n106 = Wait (ms)(milliseconds to wait=u32 100) -> (millisecond timer value=w197:u32)
            n107 = case shown="True" w198 {
              tunnel: w197 -> [_ _]
              frame False {
              }
              frame True {
                n108 = property on="program path" class="Path"() -> ("Value"=w201:path)  [unwired: 2 in, 2 out]
                n109 = property on="output filename" class="Str"() -> ("Value"=w202:string)  [unwired: 2 in, 2 out]
                n110 = Build Path(base path=w201, name or relative path=w202) -> (appended path=w200:path)
                n111 = Open/Create/Replace File(file path (use dialog)=w200, operation (0:open)=T11."replace or create") -> (refnum out=w204:refnum<file>, error out=w203:errorcluster)  [unwired: 4 in, 1 out]
                n112 = property on="configuration" class="Str"() -> ("Value"=w199:string)  [unwired: 2 in, 2 out]
                n113 = Write to Text File(file (use dialog)=w204, text=w199, error in=w203) -> (refnum out=w207:refnum<file>, error out=w206:errorcluster)  [unwired: 1 in, 1 out]
                n114 = property on="output" class="Bool (strict)"("Value"=FALSE) -> ()  [unwired: 2 in, 2 out]
                n115 = Close File(refnum=w207, error in=w206) -> ()  [unwired: 2 out]
              }
            }
          }
        }
      }
      event "file cluster.Load", "file cluster.Save", "file cluster.Saved Configuration", "file cluster.open program folder": Value Change {
        n116 = event-data() -> ()  [unwired: 1 in, 6 out]
        n117 = Wait (ms)(milliseconds to wait=u32 100) -> (millisecond timer value=w210:u32)
        n118 = flat-sequence {
          tunnel: w210 -> [_]
          frame #0 {
            n119 = property on="Saved Configuration" class="CmbBox"() -> ("Value"=w215:string)  [unwired: 2 in, 2 out]
            n120 = property on="open program folder" class="Bool (strict)"() -> ("Value"=w212:bool)  [unwired: 2 in, 2 out]
            n121 = property on="program path" class="Path"() -> ("Value"=w216:path)  [unwired: 2 in, 2 out]
            n122 = case shown="True" w212 {
              frame False {
              }
              frame True {
                n123 = property on="program path" class="Path"() -> ("Value"=w225:path)  [unwired: 2 in, 2 out]
                n124 = Path To String(path=w225) -> (string=w226:string)
                n125 = property on="open program folder" class="Bool (strict)"("Value"=FALSE) -> ()  [unwired: 2 in, 2 out]
                n126 = Concatenate Strings("explorer.exe /n /root, " ("string"), w226) -> (w227:string)
                n127 = call <vilib>:"System Exec.vi"("command line"=w227) -> ()  [unwired: 7 in, 4 out]
              }
            }
            n128 = Concatenate Strings(w215, ".dec" ("string")) -> (w221:string)
            n129 = Build Path(base path=w216, name or relative path=w221) -> (appended path=w217:path)
            n130 = List Folder(path=w216, pattern="*.dec") -> (filenames=w220:string[])  [unwired: 2 in, 3 out]
            n131 = for {
              tunnel: w220 -> [w231] mode=indexing
              tunnel: [w230] -> w219 mode=indexing
              n132 = Search/Split String(string=w231, search string/char (-)=".") -> (substring before match=w230:string)  [unwired: 1 in, 2 out]
            }
            n133 = property on="Saved Configuration" class="CmbBox"("Strings[]"=w219) -> ()  [unwired: 2 in, 2 out]
            n134 = property on="Save" class="Bool (strict)"() -> ("Value"=w213:bool)  [unwired: 2 in, 2 out]
            n135 = property on="saved controls" class="Arr (strict)"() -> ("Value"=w218:string[])  [unwired: 2 in, 2 out]
            n136 = case shown="True" w213 {
              tunnel: w218 -> [_ w241]
              tunnel: w217 -> [_ w240]
              frame False {
              }
              frame True {
                n137 = control-ref of="This VI"() -> (w243:refnum<vi>)
                n138 = call "front_panel_ctl_save.vi"("VI in"=w243, "method"=enum16{"read controls", "write controls"}."write controls", "filename"=w240, "controls"=w241) -> ("error out"=w238:errorcluster)  [unwired: 4 in]
                n139 = call <vilib>:"Clear Errors.vi"("error in (no error)"=w238) -> ()  [unwired: 5 in, 2 out]
                n140 = property on="Save" class="Bool (strict)"("Value"=FALSE) -> ()  [unwired: 2 in, 2 out]
              }
            }
            n141 = property on="Load" class="Bool (strict)"() -> ("Value"=w214:bool)  [unwired: 2 in, 2 out]
            n142 = case shown="True" w214 {
              tunnel: w218 -> [_ w234]
              tunnel: w217 -> [_ w235]
              frame False {
              }
              frame True {
                n143 = control-ref of="This VI"() -> (w236:refnum<vi>)
                n144 = call "front_panel_ctl_save.vi"("VI in"=w236, "method"=enum16{"read controls", "write controls"}."read controls", "filename"=w235, "controls"=w234) -> ("error out"=w232:errorcluster)  [unwired: 4 in]
                n145 = call <vilib>:"Clear Errors.vi"("error in (no error)"=w232) -> ()  [unwired: 5 in, 2 out]
                n146 = property on="Load" class="Bool (strict)"("Value"=FALSE) -> ()  [unwired: 2 in, 2 out]
              }
            }
          }
        }
        n147 = property on="Tab Control" class="TabCtl (strict)"() -> ("Value"=w209:T2)  [unwired: 2 in, 2 out]
        n148 = property on="Tab Control" class="TabCtl (strict)"("Val(Sgnl)"=w209) -> ()  [unwired: 2 in, 2 out]
      }
    }
  }
